vi "Write I16 as Numeric.vi"(8 "error in (no error)":errorcluster, 9 "Numeric":i16, 10 "Tag":string, 11 "Omni_Bus in":refnum<class "Omni_Bus.lvclass">) -> (0 "error out":errorcluster, 3 "Omni_Bus out":refnum<class "Omni_Bus.lvclass">)   [LabVIEW 2021, in "Omni_Bus.lvclass"]
uses:
  Omni_Bus.lvclass
  <vilib>/TSA/Abstract Data Classes/Abs_Types/Numeric/Abs_Numeric.lvclass
  C:/Program Files (x86)/National Instruments/LabVIEW 2021/vi.lib/TSA/Abstract Data Classes/Abs_Types/Type/Abs_Type.lvclass
  <vilib>/TSA/Abstract Data Classes/Abs_Types/Type/Abs_Type.lvclass/Abs_Type.ctl
  Omni_Bus.lvclass/Omni_Bus.ctl
  <vilib>/Utility/error.llb/Clear Errors.vi
  Properties/Read Var Map.vi
  <vilib>/TSA/Abstract Data Classes/Abs_Types/Type/Properties/Read Tag.vi
  <vilib>/TSA/Abstract Data Classes/Abs_Types/Value/Abs_Value.lvclass
  Check For Read Only Error.vi
  Incorrect Tag String Error.vi
  <vilib>/TSA/Abstract Data Classes/Abs_Types/Type/Abs_Type.lvclass
  C:/Program Files (x86)/National Instruments/LabVIEW 2021/vi.lib/TSA/Abstract Data Classes/Abs_Types/Value/Abs_Value.lvclass
  C:/Program Files (x86)/National Instruments/LabVIEW 2021/vi.lib/TSA/Abstract Data Classes/Abs_Types/Numeric/Abs_Numeric.lvclass
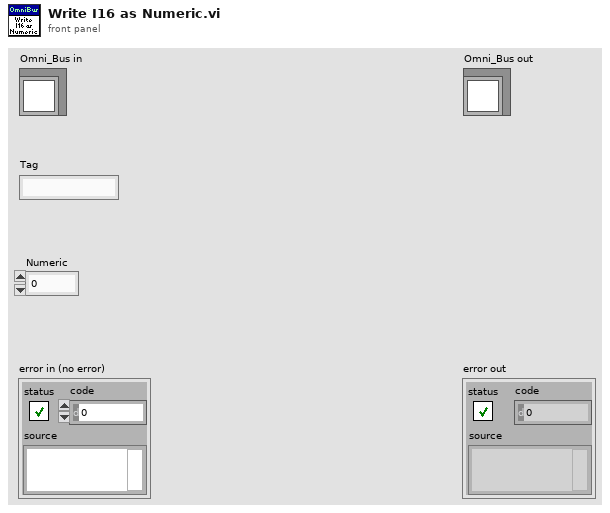
[diagram p1: front panel]
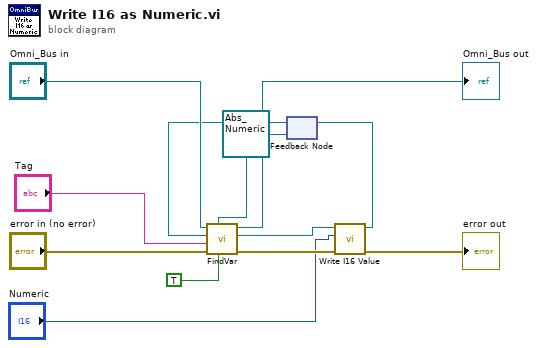
[diagram p0: block diagram]
diagram:
  w1 = refnum<class "Abs_Numeric.lvclass"> refnum ("Numeric out")
  n1 = feedback #1(w1) -> (w4:refnum<class "Abs_Numeric.lvclass">)
  n2 = call "FindVar.vi"("Write?"=TRUE, "Abs_Type"=w1, "error in (no error)"="error in (no error)", "Tag"="Tag", "Abs_Type Default"=w4, "Var Bus in"="Omni_Bus in") -> ("error out"=w8:errorcluster, "Abs_Type Found"=w5:refnum<class "Abs_Numeric.lvclass">, "Var Bus out"=→"Omni_Bus out":refnum<class "Omni_Bus.lvclass">)  [unwired: 2 in, 1 out]
  n3 = call-dynamic "Write I16 Value.vi"("error in (no error)"=w8, "I16"="Numeric", "Numeric in"=w5) -> ("error out"=→"error out":errorcluster, "Numeric out"=w6:refnum<class "Abs_Numeric.lvclass">)  [unwired: 7 in]
  n4 = feedback-in #1(w6) -> ()
